vi "GateTimeF2.vi"(8 "error in":errorcluster, 9 "stop (F)":bool) -> (0 "error out":errorcluster, 1 "Czas impulsu":dbl)   [LabVIEW 2021]
panel:
  out "stopped":bool
  in  "number of samples":i32=100
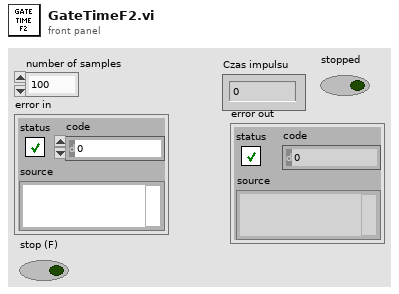
[diagram p1: front panel]
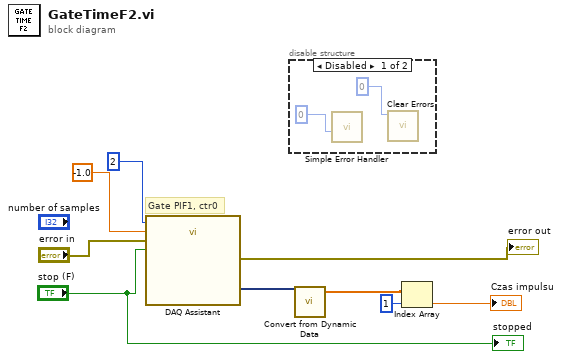
[diagram p0: block diagram]
diagram:
  # "Gate PIF1, ctr0"
  n1 = call "DAQ Assistant"("number of samples"=2, "timeout (s)"=-1.0, "error in"="error in", "stop (T)"="stop (F)") -> ("data"=w9:dynamicdata, "error out"=→"error out":errorcluster)  [unwired: 13 in, 1 out]
  n2 = disable-structure shown="Disabled" {
    frame Disabled {
      n3 = call <vilib>:"Simple Error Handler.vi"("type of dialog (OK msg:1)"=0) -> ()  [unwired: 4 in, 5 out]
      n4 = call <vilib>:"Clear Errors.vi"("specific error code to clear (0: all)"=0) -> ()  [unwired: 5 in, 2 out]
    }
    frame Enabled {
    }
  }
  n5 = call "Convert from Dynamic Data"("Dynamic Data Type"=w9) -> ("Array"=w6:dbl[])  [unwired: 3 in]
  n6 = Index Array(array=w6, index=1) -> (element=→"Czas impulsu":dbl)
  "stopped" <- "stop (F)"
